vi "controlAQuadBOutClock.vi"(7 "Set":bool, 8 "error in":errorcluster, 9 "clock in":i32, 10 "axis in":u8, 11 "connection ID":i32) -> (0 "error out":errorcluster, 1 "clock out":i32, 2 "axis out":u8, 3 "connection ID":i32)   [LabVIEW 2016]
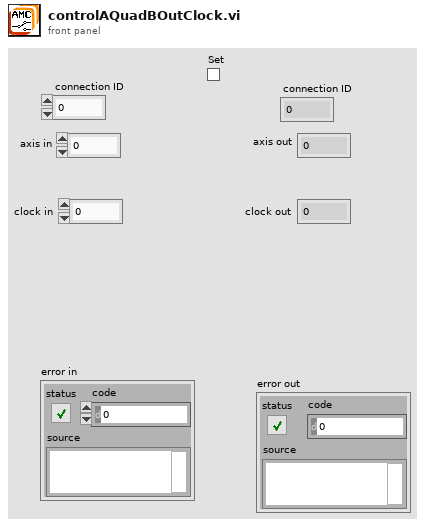
[diagram p1: front panel]
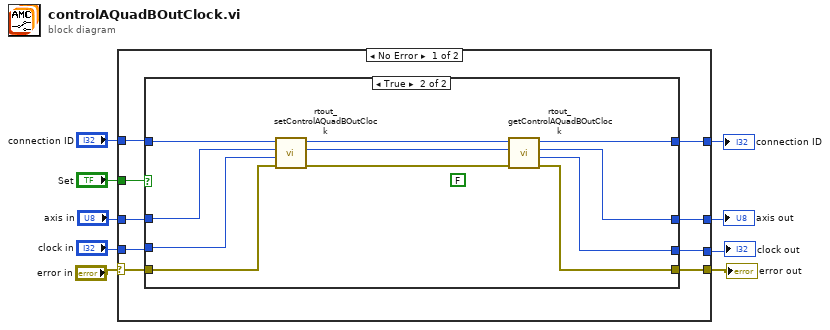
[diagram p0: block diagram]
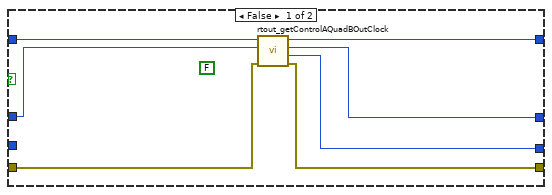
[diagram p2: hidden frame]
diagram:
  n1 = case shown="No Error" "error in" {
    selector: "error in" -> [w10 w39]
    tunnel: "axis in" -> [w16 w38]
    tunnel: [w11 w39] -> w8
    tunnel: [w15 w38] -> w7
    tunnel: "Set" -> [w14 _]
    tunnel: [w17 w37] -> w5
    tunnel: "connection ID" -> [w18 w37]
    tunnel: "clock in" -> [w12 w40]
    tunnel: [w13 w40] -> w2
    frame No Error {
      n2 = case shown="True" w14 {
        tunnel: [w23 w31] -> w17
        tunnel: w18 -> [w24 w36]
        tunnel: w16 -> [w25 w34]
        tunnel: [w19 w28] -> w15
        tunnel: [w20 w29] -> w13
        tunnel: [w21 w30] -> w11
        tunnel: w12 -> [_ w33]
        tunnel: w10 -> [w22 w35]
        frame False {
          (unwired) FALSE ("tempvalue")
          n3 = call "rtout_getControlAQuadBOutClock.vi"("error in"=w22, "axis"=w25, "connection ID"=w24) -> ("error out"=w21:errorcluster, "clock_in_ns"=w20:i32, "axis_out"=w19:i32, "connection ID"=w23:i32)  [unwired: 5 in]
        }
        frame True {
          (unwired) FALSE ("tempvalue")
          n4 = call "rtout_setControlAQuadBOutClock.vi"("error in"=w35, "clock"=w33, "axis"=w34, "connection ID"=w36) -> ("error out"=w26:errorcluster, "axis_out"=w27:i32, "connection ID"=w32:i32)  [unwired: 5 in]
          n5 = call "rtout_getControlAQuadBOutClock.vi"("error in"=w26, "axis"=w27, "connection ID"=w32) -> ("error out"=w30:errorcluster, "clock_in_ns"=w29:i32, "axis_out"=w28:i32, "connection ID"=w31:i32)  [unwired: 5 in]
        }
      }
    }
    frame Error {
    }
  }
  "error out" <- w8
  "axis out" <- w7
  "connection ID" <- w5
  "clock out" <- w2
